vi "Write Sine.vi"(8 "error in (no error)":errorcluster, 10 "Sine":dbl[](array[numeric]), 11 "NI-Scope Lock-in Driver in":refnum<class "NI-Scope Lock-in Driver.lvclass">) -> (0 "error out":errorcluster, 3 "NI-Scope Lock-in Driver out":refnum<class "NI-Scope Lock-in Driver.lvclass">)   [LabVIEW 2016, in "NI-Scope Lock-in Driver.lvclass"]
uses:
  NI-Scope Lock-in Driver.lvclass
  NI-Scope Lock-in Driver.lvclass/NI-Scope Lock-in Driver.ctl
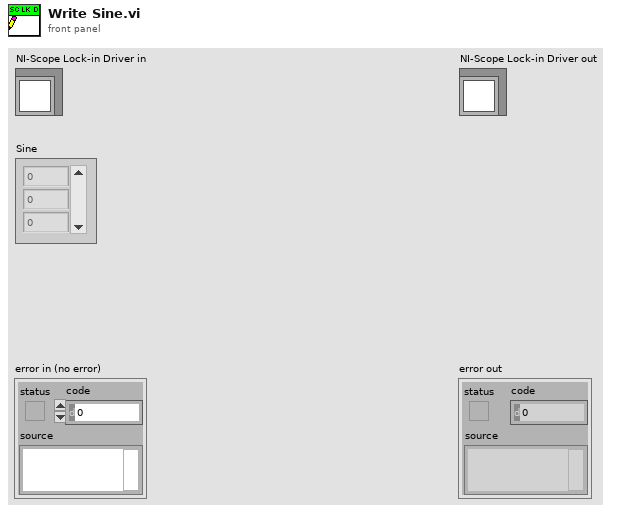
[diagram p1: front panel]
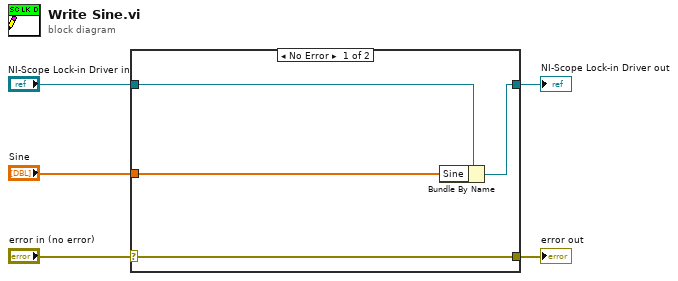
[diagram p0: block diagram]
diagram:
  n1 = case shown="No Error" "error in (no error)" {
    selector: "error in (no error)" -> [w9 w10]
    tunnel: [w9 w10] -> w4
    tunnel: [w7 w11] -> w2
    tunnel: "NI-Scope Lock-in Driver in" -> [w8 w11]
    tunnel: "Sine" -> [w6 _]
    frame No Error {
      n2 = Bundle By Name(cluster=w8, "Sine"=w6) -> (w7:refnum<class "NI-Scope Lock-in Driver.lvclass">)
    }
    frame Error {
    }
  }
  "error out" <- w4
  "NI-Scope Lock-in Driver out" <- w2
